vi "accumulate intrinsic parameters.vi"(6 "reset fixed parameters?":bool, 7 "use fixed parameters?":bool, 10 "accumulate fixed parameters":bool, 11 "fit parameters":T2) -> (1 "intrinsic parameters":T1, 3 "fixed parameter input to ftter":T2)   [LabVIEW 2017]
uses:
  typedefs/orbit parameters full.ctl
  <vilib>/ptbypt/NI_PtbyPt.lvlib
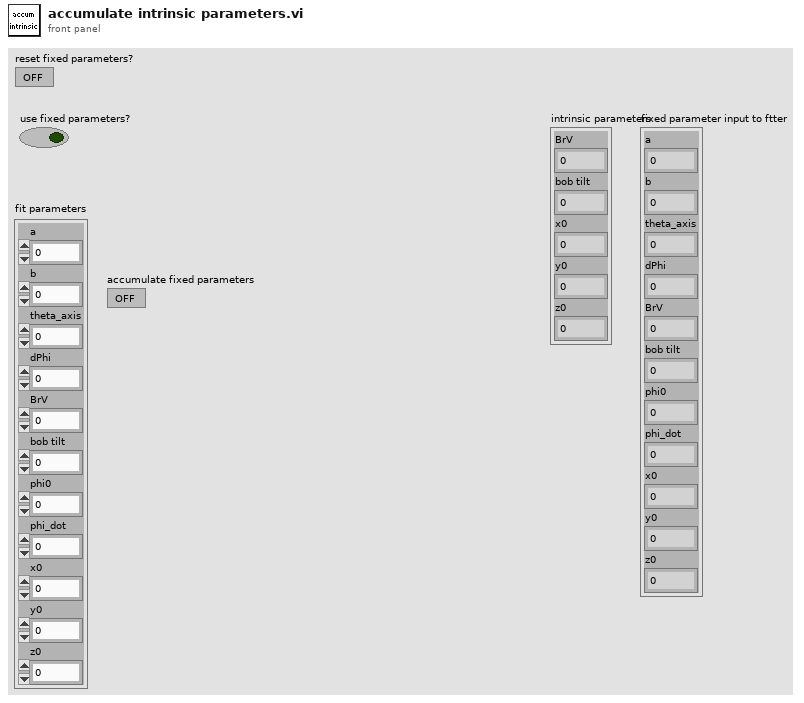
[diagram p1: front panel]
types:
  T1 = cluster{"BrV":dbl, "bob tilt":dbl, "x0":dbl, "y0":dbl, "z0":dbl}
  T2 = typedef "orbit parameters full.ctl" = cluster{"a":dbl, "b":dbl, "theta_axis":dbl, "dPhi":dbl, "BrV":dbl, "bob tilt":dbl, "phi0":dbl, "phi_dot":dbl, "x0":dbl, "y0":dbl, "z0":dbl}
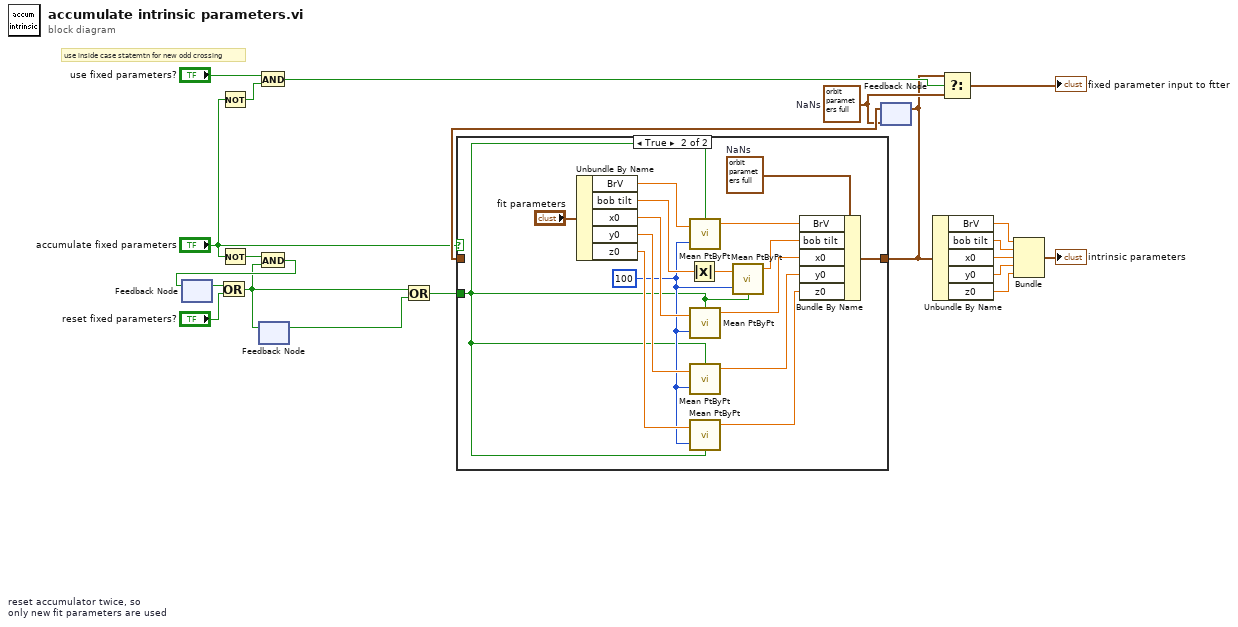
[diagram p0: block diagram]
diagram:
  w18 = T2 {"a"=nan, "b"=nan, "theta_axis"=nan, "dPhi"=nan, "BrV"=nan, "bob tilt"=nan, "phi0"=nan, "phi_dot"=nan, "x0"=nan, "y0"=nan, "z0"=nan}  # NaNs
  # "use inside case statemtn for new odd crossing"
  n1 = feedback #1() -> (w9:bool)  [unwired: 1 in]
  n2 = Or(x=w9, y="reset fixed parameters?") -> (x .or. y?=w1:bool)
  n3 = Not(x="accumulate fixed parameters") -> (.not. x?=w20:bool)
  n4 = Not(x="accumulate fixed parameters") -> (.not. x?=w6:bool)
  n5 = And(x="use fixed parameters?", y=w20) -> (x .and. y?=w19:bool)
  n6 = And(x=w6, y=w1) -> (x .and. y?=w3:bool)
  n7 = feedback-in #1(w3) -> ()
  n8 = feedback-in #2(w1) -> ()
  n9 = feedback #2 "reset accumulator twice, so \nonly new fit parameters are used"() -> (w4:bool)  [unwired: 1 in]
  n10 = Or(x=w1, y=w4) -> (x .or. y?=w2:bool)
  n11 = feedback #3(w18) -> (w21:T2)
  n12 = case shown="True" "accumulate fixed parameters" {
    tunnel: [w22 w24] -> w16
    tunnel: w21 -> [w22 _]
    tunnel: w2 -> [_ w23]
    frame False {
    }
    frame True {
      w31 = 100 ("number to average")
      w25 = T2 {"a"=nan, "b"=nan, "theta_axis"=nan, "dPhi"=nan, "BrV"=nan, "bob tilt"=nan, "phi0"=nan, "phi_dot"=nan, "x0"=nan, "y0"=nan, "z0"=nan}  # NaNs
      n13 = Unbundle By Name("fit parameters") -> ("BrV"=w35:dbl, "bob tilt"=w37:dbl, "x0"=w34:dbl, "y0"=w33:dbl, "z0"=w32:dbl)
      n14 = Absolute Value(x=w37) -> (abs(x)=w36:dbl)
      n15 = call <vilib>:"Mean PtByPt.vi"("x"=w35, "sample length"=w31, "initialize"=w23) -> ("mean"=w26:dbl)  [unwired: 1 in, 1 out]
      n16 = call <vilib>:"Mean PtByPt.vi"("x"=w34, "sample length"=w31, "initialize"=w23) -> ("mean"=w28:dbl)  [unwired: 1 in, 1 out]
      n17 = call <vilib>:"Mean PtByPt.vi"("x"=w33, "sample length"=w31, "initialize"=w23) -> ("mean"=w29:dbl)  [unwired: 1 in, 1 out]
      n18 = call <vilib>:"Mean PtByPt.vi"("x"=w32, "sample length"=w31, "initialize"=w23) -> ("mean"=w30:dbl)  [unwired: 1 in, 1 out]
      n19 = call <vilib>:"Mean PtByPt.vi"("x"=w36, "sample length"=w31, "initialize"=w23) -> ("mean"=w27:dbl)  [unwired: 1 in, 1 out]
      n20 = Bundle By Name(cluster=w25, "BrV"=w26, "bob tilt"=w27, "x0"=w28, "y0"=w29, "z0"=w30) -> (w24:T2)
    }
  }
  n21 = feedback-in #3(w16) -> ()
  n22 = Unbundle By Name(w16) -> ("BrV"=w15:dbl, "bob tilt"=w14:dbl, "x0"=w13:dbl, "y0"=w12:dbl, "z0"=w11:dbl)
  n23 = Select(t=w16, s=w19, f=w18) -> (s? t:f=→"fixed parameter input to ftter":T2)
  n24 = Bundle("BrV"=w15, "bob tilt"=w14, "x0"=w13, "y0"=w12, "z0"=w11) -> (→"intrinsic parameters":T1)  [unwired: 1 in]
